vi "Initialize UI.vi"(8 "error in (no error)":errorcluster, 10 "Control Refs":T2, 11 "node ref in":T1) -> (0 "error out":errorcluster, 2 "Linux?":bool, 3 "node ref out":T1)   [LabVIEW 2015, in "TDMS datalogger editor node.lvclass"]
uses:
  TDMS datalogger editor node.lvclass
  <vilib>/NI/Configuration Framework/Node/NodeRef.ctl
  <vilib>/NI/Configuration Framework/Node/NISE_CEF_Node.lvclass
  Control Refs.ctl
  module/configuration/TDMS datalogger configuration.lvclass
  TDMS datalogger editor node.lvclass/TDMS datalogger editor node.ctl
  module/configuration/TDMS datalogger configuration.lvclass/TDMS datalogger configuration.ctl
  Write channel table.vi
  Write avail tags table.vi
  module/configuration/Read backup directory.vi
  module/configuration/Read Path.vi
  module/configuration/Read queue size.vi
  module/configuration/Read scans per write.vi
  module/configuration/Read add enable channel.vi
  module/configuration/Read channel pattern matches.vi
  module/configuration/Read log name.vi
  module/configuration/Read logrotate_options.vi
  <vilib>/NI/DCAF/Tag Editor Core/Configuration Editor/Classes/Module editor node/Read Module Configuration.vi
  <vilib>/NI/Tag Bus Module Framework/module configuration/TBM module configuration.lvclass
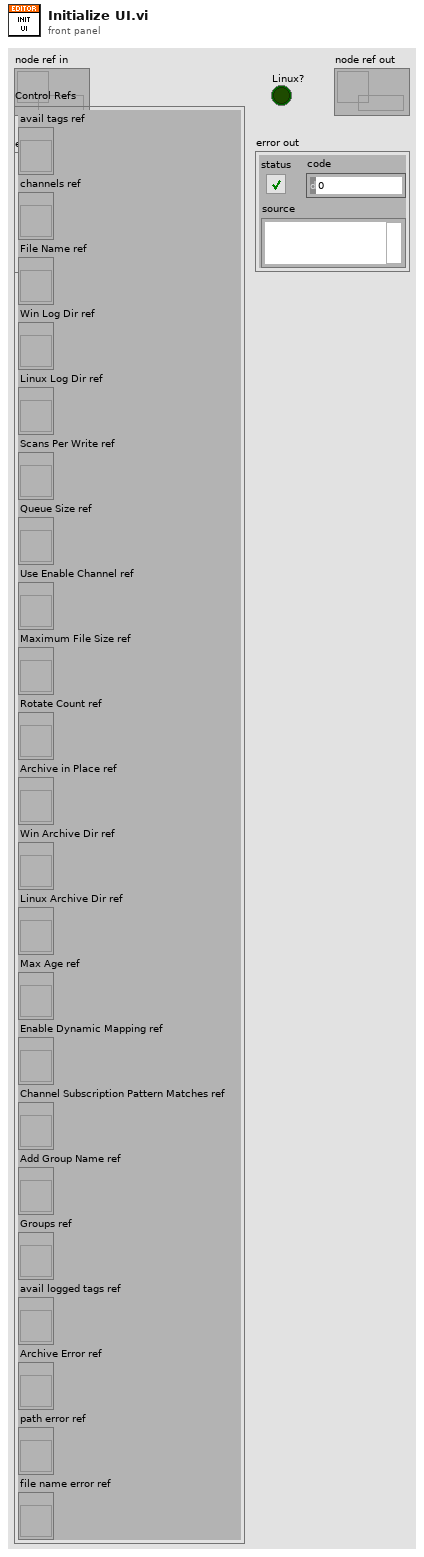
[diagram p1: front panel]
types:
  T1 = typedef "NISE_CEF_Node.lvclass/NodeRef.ctl" = refnum<data-value>
  T2 = typedef "Control Refs.ctl" = cluster{"avail tags ref":refnum<vi>, "channels ref":refnum<vi>, "File Name ref":refnum<vi>, "Win Log Dir ref":refnum<vi>, "Linux Log Dir ref":refnum<vi>, "Scans Per Write ref":refnum<vi>, "Queue Size ref":refnum<vi>, "Use Enable Channel ref":refnum<vi>, "Maximum File Size ref":refnum<vi>, "Rotate Count ref":refnum<vi>, "Archive in Place ref":refnum<vi>, "Win Archive Dir ref":refnum<vi>, "Linux Archive Dir ref":refnum<vi>, "Max Age ref":refnum<vi>, "Enable Dynamic Mapping ref":refnum<vi>, "Channel Subscription Pattern Matches ref":refnum<vi>, "Add Group Name ref":refnum<vi>, "Groups ref":refnum<vi>, "avail logged tags ref":refnum<vi>, "Archive Error ref":refnum<vi>, "path error ref":refnum<vi>, "file name error ref":refnum<vi>}
  T3 = typedef "TBM configuration.lvclass/Target Types.ctl" = enum16{"Windows", "Mac", "Linux", "Linux RT ARM", "VxWorks", "Pharlap", "Other", "Linux RT x64"}
  T4 = typedef "LogRotate.lvclass/options.ctl" = cluster{"max file size (bytes)":i64, "rotate count":u32, "max age (days)":dbl, "No archive dir":bool, "Archive dir":path}
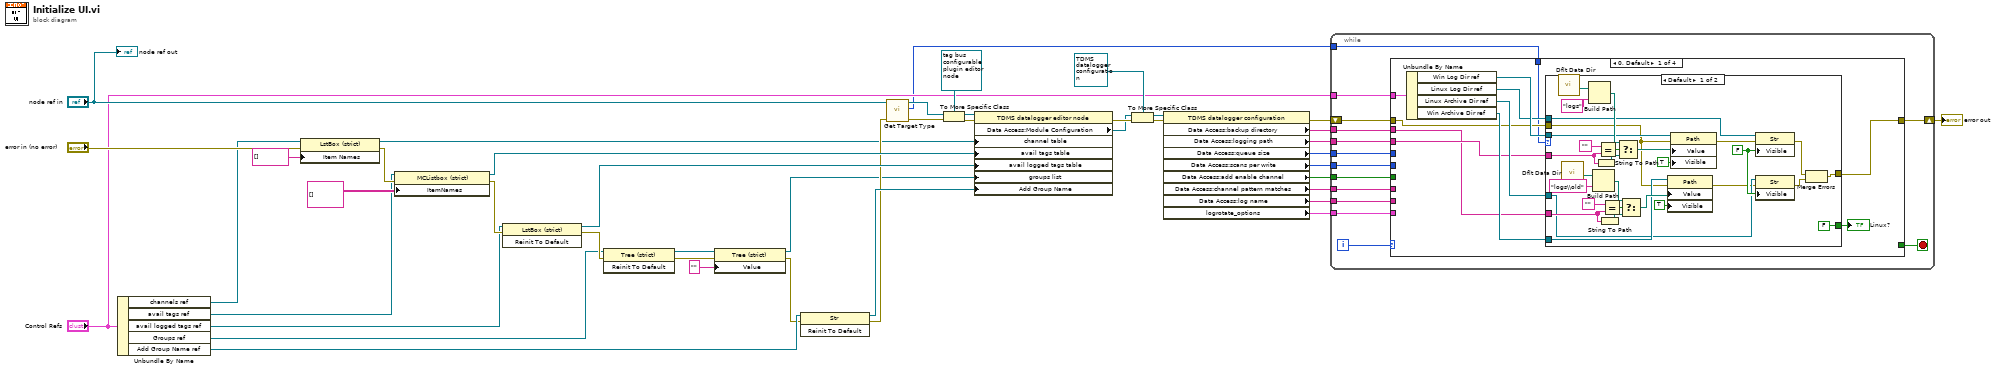
[diagram p0: block diagram]
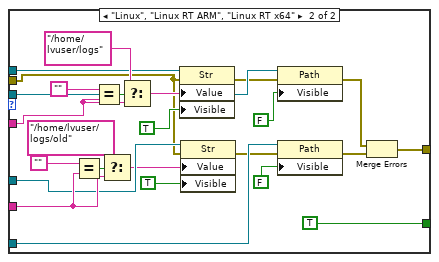
[diagram p2: hidden frame]
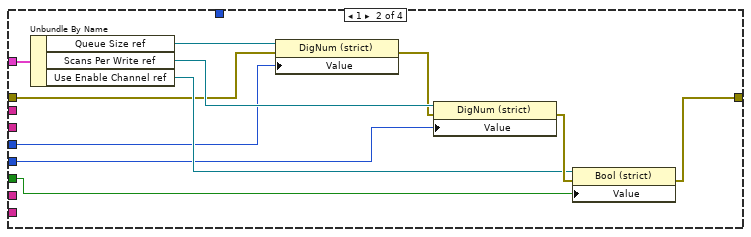
[diagram p3: hidden frame]
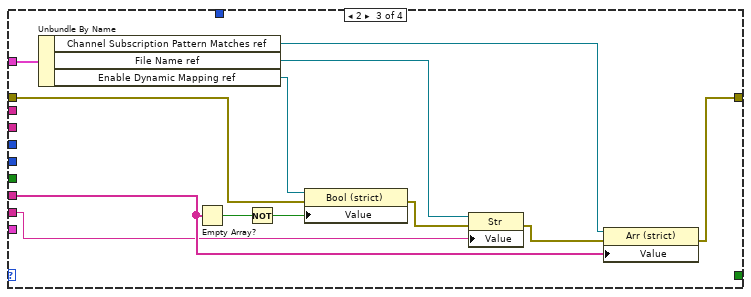
[diagram p4: hidden frame]
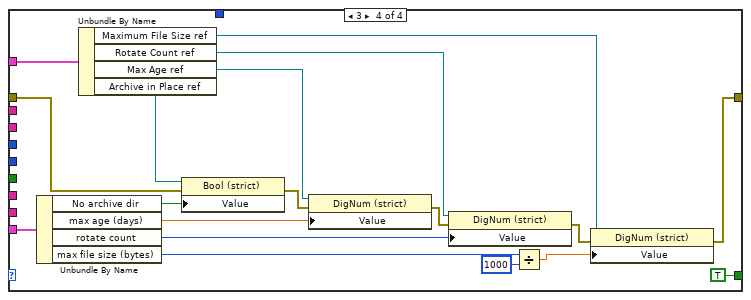
[diagram p5: hidden frame]
diagram:
  n1 = Unbundle By Name("Control Refs") -> ("channels ref"=w22:refnum<vi>, "avail tags ref"=w21:refnum<vi>, "avail logged tags ref"=w20:refnum<vi>, "Groups ref"=w19:refnum<vi>, "Add Group Name ref"=w18:refnum<vi>)
  n2 = property on="Property Node" class="LstBox (strict)"(reference=w22, error in="error in (no error)", "Item Names"=string[] []) -> (reference out=w17:refnum<vi>, error out=w27:errorcluster)
  n3 = property on="Property Node" class="MCListbox (strict)"(reference=w21, error in=w27, "ItemNames"=string[][] [] ("Item Names")) -> (reference out=w29:refnum<vi>, error out=w26:errorcluster)
  n4 = invoke class="LstBox (strict)" method="Reinit To Default"(reference=w20, error in=w26) -> (reference out=w30:refnum<vi>, error out=w25:errorcluster)  [unwired: 1 in, 1 out]
  n5 = invoke class="Tree (strict)" method="Reinit To Default"(reference=w19, error in=w25) -> (reference out=w15:refnum<vi>, error out=w16:errorcluster)  [unwired: 1 in, 1 out]
  n6 = property on="Property Node" class="Tree (strict)"(reference=w15, error in=w16, "Value"="" ("Groups")) -> (reference out=w14:refnum<vi>, error out=w13:errorcluster)
  n7 = invoke class="Str" method="Reinit To Default"(reference=w18, error in=w13) -> (reference out=w28:refnum<vi>, error out=w24:errorcluster)  [unwired: 1 in, 1 out]
  n8 = call "Get Target Type.vi"("error in (no error)"=w24, "node ref in"="node ref in") -> ("error out"=w34:errorcluster, "Target Type"=w8:T3, "node ref out"=w33:T1)  [unwired: 6 in]
  n9 = To More Specific Class(target class=refnum<data-value> refnum ("data value reference"), reference=w33, error in=w34) -> (specific class reference=w37:refnum<data-value>, error out=w36:errorcluster)
  n10 = property class="TDMS datalogger editor node"(reference=w37, error in=w36, "channel table"=w17, "avail tags table"=w29, "avail logged tags table"=w30, "groups list"=w14, "Add Group Name"=w28) -> (error out=w44:errorcluster, "Data Access:Module Configuration"=w42:refnum<class "TBM module configuration.lvclass">)  [unwired: 1 out]
  n11 = To More Specific Class(target class=refnum<class "TDMS datalogger configuration.lvclass"> refnum ("TDMS datalogger configuration"), reference=w42, error in=w44) -> (specific class reference=w40:refnum<class "TDMS datalogger configuration.lvclass">, error out=w43:errorcluster)
  n12 = property class="TDMS datalogger configuration"(reference=w40, error in=w43) -> (error out=w9:errorcluster, "Data Access:backup directory"=w10:string, "Data Access:logging path"=w11:string, "Data Access:queue size"=w7:u16, "Data Access:scans per write"=w5:u16, "Data Access:add enable channel"=w6:bool, "Data Access:channel pattern matches"=w4:string[], "Data Access:log name"=w3:string, "logrotate_options"=w2:T4)  [unwired: 1 out]
  n13 = while {
    tunnel: "Control Refs" -> [w56]
    tunnel: w11 -> [w55]
    tunnel: w10 -> [w54]
    shift-right: [w53] -> w1
    shift-left: w9 -> [w52]
    tunnel: w8 -> [w51]
    tunnel: w7 -> [w50]
    tunnel: w5 -> [w49]
    tunnel: w6 -> [w48]
    tunnel: w4 -> [w47]
    tunnel: w3 -> [w46]
    tunnel: w2 -> [w45]
    i -> [w57]
    stop <- w58 stop-if-true
    n14 = case shown="0, Default" w57 {
      tunnel: [_ _ _ TRUE] -> w58
      tunnel: w56 -> [w69 w135 w145 w163]
      tunnel: w55 -> [w63 _ _ _]
      tunnel: w54 -> [w62 _ _ _]
      tunnel: [w61 w125 w136 w151] -> w53
      tunnel: w52 -> [w60 w126 w139 w152]
      tunnel: w51 -> [w59 _ _ _]
      tunnel: w50 -> [_ w129 _ _]
      tunnel: w49 -> [_ w128 _ _]
      tunnel: w48 -> [_ w127 _ _]
      tunnel: w47 -> [_ _ w141 _]
      tunnel: w46 -> [_ _ w140 _]
      tunnel: w45 -> [_ _ _ w165]
      frame 0, Default {
        n15 = Unbundle By Name(w69) -> ("Win Log Dir ref"=w67:refnum<vi>, "Linux Log Dir ref"=w66:refnum<vi>, "Linux Archive Dir ref"=w64:refnum<vi>, "Win Archive Dir ref"=w65:refnum<vi>)
        n16 = case shown="Default" w59 {
          tunnel: w62 -> [w81 w111]
          tunnel: w63 -> [w90 w117]
          tunnel: [FALSE TRUE] -> w68
          tunnel: w66 -> [w78 w110]
          tunnel: w64 -> [w76 w109]
          tunnel: w67 -> [w79 w108]
          tunnel: w65 -> [w77 w107]
          tunnel: [w73 w102] -> w61
          tunnel: w60 -> [w70 w100]
          frame Default {
            w97 = FALSE ("Visible")
            n17 = call <vilib>:"Dflt Data Dir.vi"() -> ("App:Default Data Directory"=w93:path)
            n18 = call <vilib>:"Dflt Data Dir.vi"() -> ("App:Default Data Directory"=w84:path)
            n19 = Build Path(base path=w93, name or relative path="logs") -> (appended path=w95:path)
            n20 = Build Path(base path=w84, name or relative path="logs\\old") -> (appended path=w82:path)
            n21 = String To Path(string=w90) -> (path=w89:path)
            n22 = Equal?(x="", y=w90) -> (x = y?=w91:bool)
            n23 = String To Path(string=w81) -> (path=w87:path)
            n24 = Equal?(x="", y=w81) -> (x = y?=w86:bool)
            n25 = Select(t=w95, s=w91, f=w89) -> (s? t:f=w88:path)
            n26 = Select(t=w82, s=w86, f=w87) -> (s? t:f=w80:path)
            n27 = property on="Property Node" class="Path"(reference=w77, error in=w70, "Value"=w80, "Visible"=TRUE) -> (error out=w75:errorcluster)  [unwired: 1 out]
            n28 = property on="Property Node" class="Path"(reference=w79, error in=w70, "Value"=w88, "Visible"=TRUE) -> (error out=w71:errorcluster)  [unwired: 1 out]
            n29 = property on="Property Node" class="Str"(reference=w78, error in=w71, "Visible"=w97) -> (error out=w72:errorcluster)  [unwired: 1 out]
            n30 = property on="Property Node" class="Str"(reference=w76, error in=w75, "Visible"=w97) -> (error out=w74:errorcluster)  [unwired: 1 out]
            n31 = Merge Errors(w72, w74) -> (w73:errorcluster)
          }
          frame "Linux", "Linux RT ARM", "Linux RT x64" {
            n32 = Equal?(x="", y=w111) -> (x = y?=w113:bool)
            n33 = Equal?(x="", y=w117) -> (x = y?=w118:bool)
            n34 = Select(t="/home/lvuser/logs/old", s=w113, f=w111) -> (s? t:f=w106:string)
            n35 = Select(t="/home/lvuser/logs", s=w118, f=w117) -> (s? t:f=w116:string)
            n36 = property on="Property Node" class="Str"(reference=w110, error in=w100, "Value"=w116, "Visible"=TRUE) -> (error out=w104:errorcluster)  [unwired: 1 out]
            n37 = property on="Property Node" class="Str"(reference=w109, error in=w100, "Value"=w106, "Visible"=TRUE) -> (error out=w105:errorcluster)  [unwired: 1 out]
            n38 = property on="Property Node" class="Path"(reference=w108, error in=w104, "Visible"=FALSE) -> (error out=w101:errorcluster)  [unwired: 1 out]
            n39 = property on="Property Node" class="Path"(reference=w107, error in=w105, "Visible"=FALSE) -> (error out=w103:errorcluster)  [unwired: 1 out]
            n40 = Merge Errors(w101, w103) -> (w102:errorcluster)
          }
        }
        "Linux?" <- w68
      }
      frame 1 {
        n41 = Unbundle By Name(w135) -> ("Queue Size ref"=w134:refnum<vi>, "Scans Per Write ref"=w133:refnum<vi>, "Use Enable Channel ref"=w130:refnum<vi>)
        n42 = property on="Property Node" class="DigNum (strict)"(reference=w134, error in=w126, "Value"=w129) -> (error out=w132:errorcluster)  [unwired: 1 out]
        n43 = property class="DigNum (strict)"(reference=w133, error in=w132, "Value"=w128) -> (error out=w131:errorcluster)  [unwired: 1 out]
        n44 = property on="Property Node" class="Bool (strict)"(reference=w130, error in=w131, "Value"=w127) -> (error out=w125:errorcluster)  [unwired: 1 out]
      }
      frame 2 {
        n45 = Unbundle By Name(w145) -> ("Channel Subscription Pattern Matches ref"=w144:refnum<vi>, "File Name ref"=w143:refnum<vi>, "Enable Dynamic Mapping ref"=w142:refnum<vi>)
        n46 = Empty Array?(array=w141) -> (empty?=w146:bool)
        n47 = Not(x=w146) -> (.not. x?=w147:bool)
        n48 = property on="Property Node" class="Bool (strict)"(reference=w142, error in=w139, "Value"=w147) -> (error out=w138:errorcluster)  [unwired: 1 out]
        n49 = property on="Property Node" class="Str"(reference=w143, error in=w138, "Value"=w140) -> (error out=w137:errorcluster)  [unwired: 1 out]
        n50 = property class="Arr (strict)"(reference=w144, error in=w137, "Value"=w141) -> (error out=w136:errorcluster)  [unwired: 1 out]
      }
      frame 3 {
        n51 = Unbundle By Name(w165) -> ("No archive dir"=w155:bool, "max age (days)"=w154:dbl, "rotate count"=w153:u32, "max file size (bytes)"=w149:i64)
        n52 = Unbundle By Name(w163) -> ("Maximum File Size ref"=w162:refnum<vi>, "Rotate Count ref"=w161:refnum<vi>, "Max Age ref"=w159:refnum<vi>, "Archive in Place ref"=w157:refnum<vi>)
        n53 = property on="Property Node" class="Bool (strict)"(reference=w157, error in=w152, "Value"=w155) -> (error out=w156:errorcluster)  [unwired: 1 out]
        n54 = property on="Property Node" class="DigNum (strict)"(reference=w159, error in=w156, "Value"=w154) -> (error out=w158:errorcluster)  [unwired: 1 out]
        n55 = property on="Property Node" class="DigNum (strict)"(reference=w161, error in=w158, "Value"=w153) -> (error out=w160:errorcluster)  [unwired: 1 out]
        n56 = Divide(x=w149, y=i64 1000) -> (x/y=w148:dbl)
        n57 = property on="Property Node" class="DigNum (strict)"(reference=w162, error in=w160, "Value"=w148) -> (error out=w151:errorcluster)  [unwired: 1 out]
      }
    }
  }
  "error out" <- w1
  "node ref out" <- "node ref in"
